vi "6. SCADA_Robotic_Arm_2.vi"() -> ()   [LabVIEW 2019]
panel:
  in  "Tab Control":enum32{"Control Panel"}(tab)
  in  "LEFT/RIGHT":dbl(slide) scale=0.0..500.0
  in  "Bottle Pic":bool
  in  "UP/DOWN":dbl(slide) scale=157.0..420.0
  in  "stop":bool
  out "Boolean":bool
  out "Boolean 4":bool
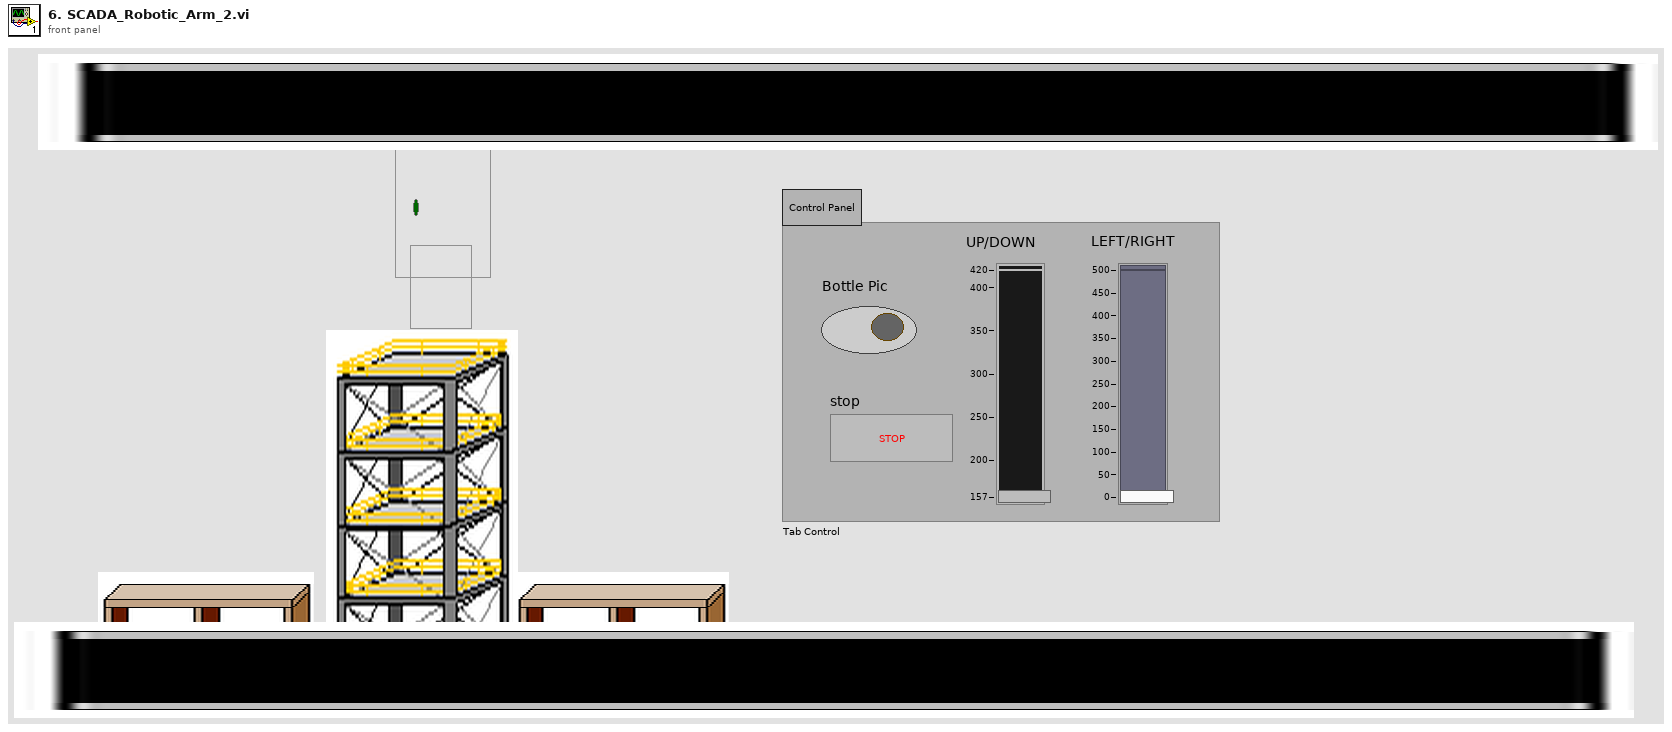
[diagram p1: front panel]
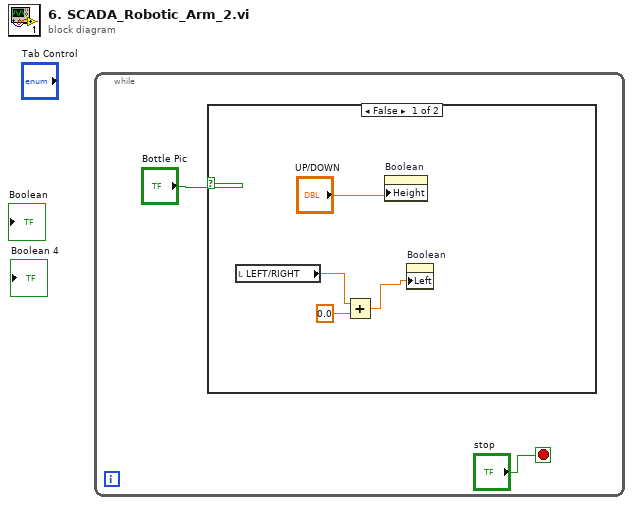
[diagram p0: block diagram]
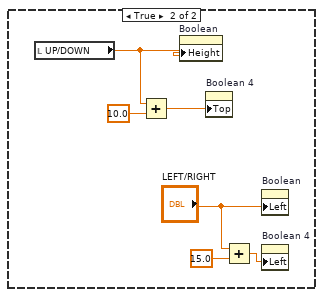
[diagram p2: hidden frame]
diagram:
  n1 = while {
    stop <- "stop" stop-if-true
    n2 = case shown="False" "Bottle Pic" {
      frame False {
        n3 = local read "LEFT/RIGHT"() -> (w4:dbl)
        n4 = Add(x=w4, y=0.0) -> (x+y=w3:dbl)
        n5 = property on="Boolean" class="Bool (strict)"("Height"="UP/DOWN") -> ()  [unwired: 2 in, 2 out]
        n6 = property on="Boolean" class="Bool (strict)"("Left"=w3) -> ()  [unwired: 2 in, 2 out]
      }
      frame True {
        n7 = local read "UP/DOWN"() -> (w12:dbl)
        n8 = Add(x=w12, y=10.0) -> (x+y=w11:dbl)
        n9 = property on="Boolean" class="Bool (strict)"("Height"=w12) -> ()  [unwired: 2 in, 2 out]
        n10 = property on="Boolean 4" class="Bool (strict)"("Top"=w11) -> ()  [unwired: 2 in, 2 out]
        n11 = Add(x="LEFT/RIGHT", y=15.0) -> (x+y=w9:dbl)
        n12 = property on="Boolean" class="Bool (strict)"("Left"="LEFT/RIGHT") -> ()  [unwired: 2 in, 2 out]
        n13 = property on="Boolean 4" class="Bool (strict)"("Left"=w9) -> ()  [unwired: 2 in, 2 out]
      }
    }
  }
